vi "Q Host Data (SubVI).vi"(8 "error in":errorcluster, 11 "IP":string) -> (0 "error out":errorcluster, 1 "# elements in queue":i32, 2 "DO Change?":bool, 3 "Data":T1)   [LabVIEW 2021]
uses:
  Controls/Host Data Cluster.ctl
  Main Engine/Controls/Main Engine CPU Info.ctl
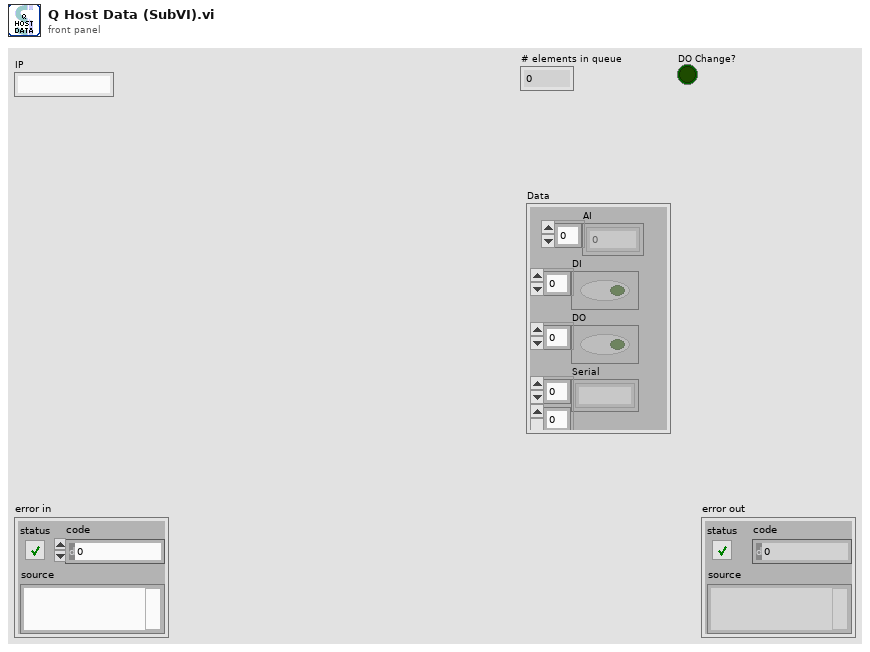
[diagram p1: front panel]
types:
  T1 = typedef "Host Data Cluster.ctl" = cluster{"AI":dbl[], "DI":bool[], "DO":bool[], "Serial":string[][], "CPU":T2, "Stop":bool, "DO Channel":string[]}
  T2 = typedef "Main Engine CPU Info.ctl" = cluster{"Total Load":u32[], "Interrupt Load":u32[], "Total Physical":dbl, "Free Physical":dbl, "Primary Disk Capacity":dbl, "Primary Disk Free":dbl}
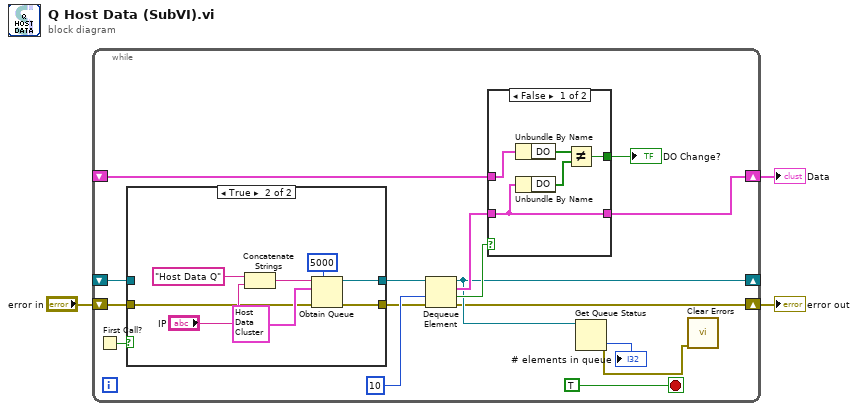
[diagram p0: block diagram]
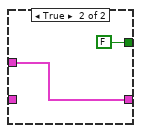
[diagram p2: hidden frame]
diagram:
  n1 = while {
    shift-right: [w5] -> _
    shift-left: _ -> [w14]
    shift-right: [w4] -> w2
    shift-left: "error in" -> [w13]
    shift-right: [w9] -> w1
    shift-left: _ -> [w11]
    stop <- TRUE stop-if-true
    n2 = First Call?() -> (First Call?: T/F=w15:bool)
    n3 = case shown="True" w15 {
      tunnel: [w28 w32] -> w18
      tunnel: [w27 w30] -> w16
      tunnel: w14 -> [w28 _]
      tunnel: w13 -> [w27 w29]
      frame False {
      }
      frame True {
        n4 = Concatenate Strings("Host Data Q" ("name (unnamed)"), "IP") -> (w34:string)
        n5 = Obtain Queue(max queue size (-1, unlimited)=5000, name (unnamed)=w34, element data type=T1 {"AI"=[-3.29963760152739, -3.28042607250678, -3.30275742266883, -3.28305329003257, -3.29914499819412, -3.27566424083626, -3.29520417157553, -3.26269235518028, -3.14446761533159, -3.13215254239399, -3.16088771377303, -3.13198834142664, -3.16959036650255, -3.151528257494, -3.17188918049567, -3.1431540075152, -3.2208210848143, -3.21425304324317, -3.24479443847459, -3.23132995179905, -3.24922786722435, -3.22706072451644, -3.22311989941762, -3.18896608529332, -3.07895143597999, -3.07616002028715, -3.11064221681751, -3.08551947305428, -3.12459929803547, -3.10916440827463, -3.12197208267327], "DI"=[FALSE, FALSE, FALSE, FALSE, FALSE, FALSE, FALSE, FALSE, FALSE, FALSE, FALSE, FALSE, FALSE, FALSE, FALSE, FALSE, FALSE, FALSE, FALSE, FALSE, FALSE, FALSE, FALSE, FALSE, FALSE, FALSE, FALSE, FALSE, FALSE, FALSE, FALSE, FALSE, FALSE, FALSE, FALSE, FALSE, FALSE, FALSE, FALSE, FALSE, FALSE, FALSE, FALSE, FALSE, FALSE, FALSE, FALSE, FALSE, FALSE, FALSE, FALSE, FALSE, FALSE, FALSE, FALSE, FALSE, FALSE, FALSE, FALSE, FALSE, FALSE, FALSE, FALSE, FALSE], "DO"=[], "Serial"=[], "CPU"={"Total Load"=[], "Interrupt Load"=[], "Total Physical"=0.0, "Free Physical"=0.0, "Primary Disk Capacity"=0.0, "Primary Disk Free"=0.0}, "Stop"=FALSE, "DO Channel"=[]} ("Data Out"), error in (no error)=w29) -> (queue out=w32:refnum<queue>, error out=w30:errorcluster)  [unwired: 1 in, 1 out]
      }
    }
    n6 = Dequeue Element(queue=w18, timeout in ms (-1)=10, error in (no error)=w16) -> (queue out=w5:refnum<queue>, element=w8:T1, timed out?=w12:bool, error out=w4:errorcluster)
    n7 = case shown="False" w12 {
      tunnel: w8 -> [w23 _]
      tunnel: [w23 w26] -> w9
      tunnel: w11 -> [w24 w26]
      tunnel: [w21 FALSE] -> w10
      frame False {
        n8 = Unbundle By Name(w24) -> ("DO"=w20:bool[])
        n9 = Unbundle By Name(w23) -> ("DO"=w22:bool[])
        n10 = Not Equal?(x=w20, y=w22) -> (x != y?=w21:bool)
      }
      frame True {
      }
    }
    "DO Change?" <- w10
    n11 = Get Queue Status(queue=w5) -> (error out=w6:errorcluster, # elements in queue=→"# elements in queue":i32)  [unwired: 2 in, 6 out]
    n12 = call <vilib>:"Clear Errors.vi"("error in (no error)"=w6) -> ()  [unwired: 5 in, 2 out]
  }
  "error out" <- w2
  "Data" <- w1
